vi "DPIO-Write Data.vi"(0 "DP stimulus params":T1={"Start (dB)"=0.0, "Stop (dB)"=0.0, "Step (dB)"=0.0, "Ear"=enum."Left", "Mode"=enum."L1 = L2", "f2 freqs (kHz)"=""}, 5 "AO Info":T3={"Samples/buffer (If continuous)"=10000, "p-p V output"=10.0, "Update Interval (uS)"=10, "# Reps"=10, "Mode"=0} {"Mode" items=["Free Run", "Set Reps", "WaveGen Only"]; "p-p V output" format="%.2f"}, 7 "DATA ARRAY TO SAVE":dbl[][](array[numeric])=[[60.0, 8337.40234375, 9997.55859375, 75.26988695602513, 60.02010719537736, -2.497224379667877, -6.035718747331266, -13.246407124310245, -10.010309675121785], [61.0, 8337.40234375, 9997.55859375, 75.26843338154123, 61.04772121995559, -10.079260881420453, -2.002824821632224, -13.478836216499538, -9.891536524361616], [62.0, 8337.40234375, 9997.55859375, 75.26842118127979, 62.07823756136253, -2.037295999935573, -2.3383554984418637, -7.356473706785984, -12.202574186674596], [63.0, 8337.40234375, 9997.55859375, 75.26689847125223, 63.11596204731964, 1.7137665521003527, -3.501789694558177, -12.430751170506419, -10.332402563871469], [64.0, 8337.40234375, 9997.55859375, 75.26410902438056, 64.14546808637438, 2.214385186705627, -2.5193547021211913, -13.192878839530465, -9.010065513616713], [65.0, 8337.40234375, 9997.55859375, 75.26244780852893, 65.23791090720081, 2.0929092941162324, -2.858976817533751, -9.447162706703264, -9.16426721329621], [66.0, 8337.40234375, 9997.55859375, 75.25853649879664, 66.25922378984633, 1.2609285848979752, -0.7601294228255071, -5.149516176783557, -11.823646373895414], [67.0, 8337.40234375, 9997.55859375, 75.25746587316436, 67.30068235725267, 2.1908463904635838, -2.0222825519681606, -4.18117048366198, -11.637986568273387], [68.0, 8337.40234375, 9997.55859375, 75.27653659482075, 68.25845427744406, -0.29516344046096776, -4.10442801745323, -4.280981245973685, -12.110717739994087], [69.0, 8337.40234375, 9997.55859375, 75.27405688750105, 69.30238527627466, -7.496556220976231, -3.7432906885060433, -6.52360859523705, -11.301872512577514], [70.0, 8337.40234375, 9997.55859375, 75.27095405136916, 70.32073725195177, -7.652753711444348, -2.8528280454442765, -12.182093372567518, -10.666926947025527], [71.0, 8337.40234375, 9997.55859375, 75.26930497101785, 71.37084081139689, -1.5072623443189102, -3.405227655422884, -9.054202292188972, -11.053257216259539], [72.0, 8337.40234375, 9997.55859375, 75.26969080860029, 72.40219775773258, -0.3774238902284708, -3.754108910689375, -6.28964062573494, -13.220161518942938], [73.0, 8337.40234375, 9997.55859375, 75.27097215908172, 73.44142356983946, -3.2633324671698247, -2.5245927600519877, -2.7612590826062373, -9.965708629780178], [74.0, 8337.40234375, 9997.55859375, 75.26718617542848, 74.4794351336158, -1.320663115916176, -4.039221123608023, -2.1363104698355713, -10.603442564638495], [75.0, 8337.40234375, 9997.55859375, 75.26504354514502, 75.52130171920129, -2.818101467950008, -3.4587578575361917, -6.091970124277275, -11.100841890245615]] format="%.2f", 9 "WAVEFORM ARRAY TO SAVE":dbl[][](array[numeric]) format="%.2f", 11 "error in (no error)":errorcluster, 12 "Averaging Specs":T4={"#Waves to Ave"=25, "#Spectra to Ave"=4}, 13 "Gain (dB)":dbl, 14 "Notes":string) -> (15 "error out":errorcluster)   [LabVIEW 2020]
uses:
  ABI Chamber VIs/LV Source/ABI Chamber Controller/SubVIs/ABI Globals.vi
  Utility VIs/Type Defs/Left-Right ring.ctl
  Typedefs/DP Stimulus Params.ctl
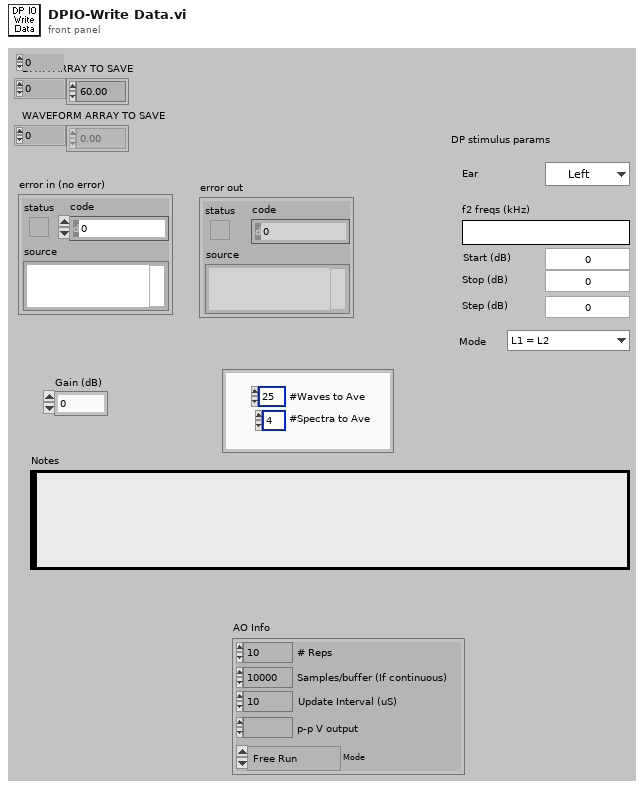
[diagram p1: front panel]
types:
  T1 = typedef "DP Stimulus Params.ctl" = cluster{"Start (dB)":dbl, "Stop (dB)":dbl, "Step (dB)":dbl, "Ear":T2, "Mode":enum16{"L1 = L2", "L1 = L2 + 10 dB"}, "f2 freqs (kHz)":string}
  T2 = typedef "Left-Right ring.ctl" = enum16{"Right", "Left"}
  T3 = cluster{"Samples/buffer (If continuous)":i32, "p-p V output":ext, "Update Interval (uS)":i32, "# Reps":i32, "Mode":u16}
  T4 = cluster{"#Waves to Ave":i32, "#Spectra to Ave":i32}
  T5 = enum16{"open", "replace", "create", "open or create", "replace or create", "replace or create with confirmation"}
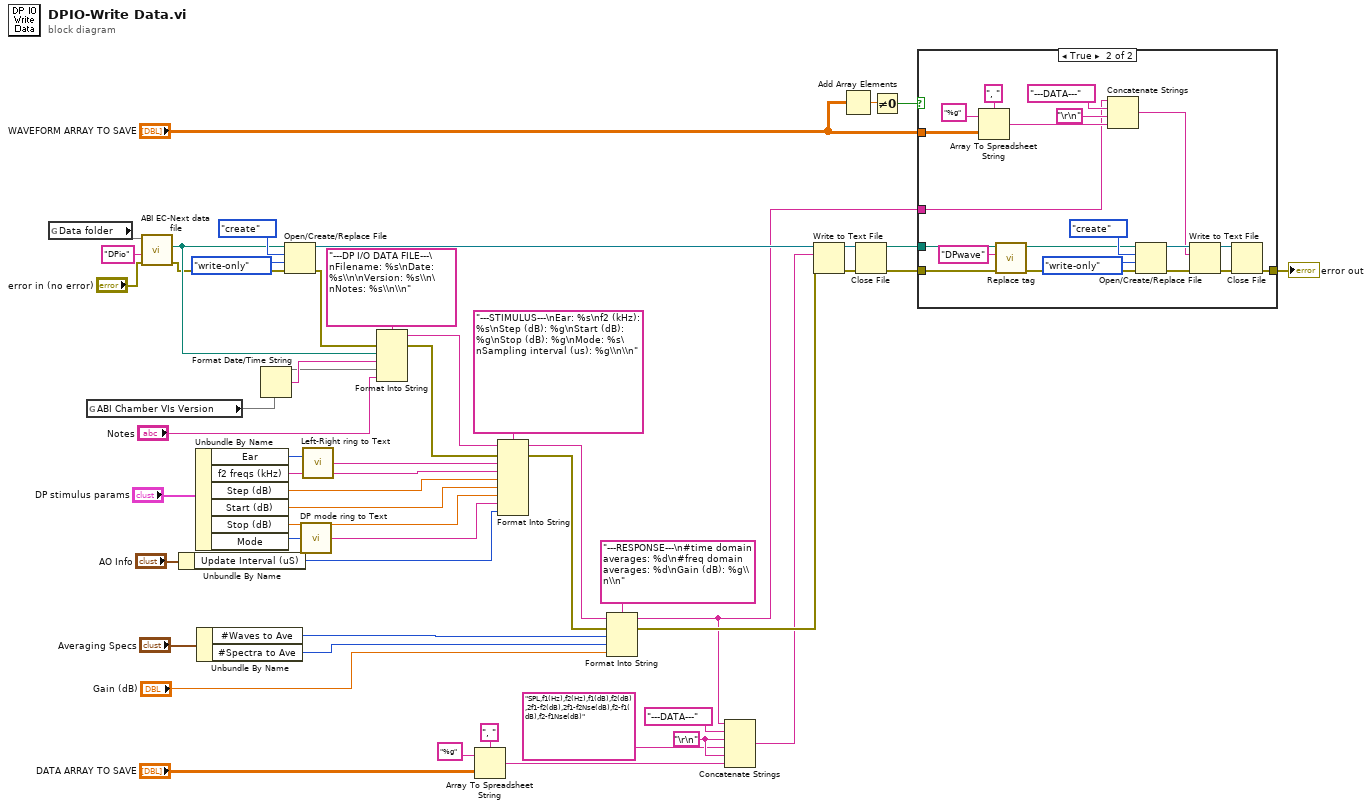
[diagram p0: block diagram]
diagram:
  w18 = "\r\n"
  n1 = global read "ABI Globals.vi" "Data folder"() -> (w15)
  n2 = global read "ABI Globals.vi" "ABI Chamber VIs Version"() -> (w31)
  n3 = call "ABI EC-Next data file.vi"("error in (no error)"="error in (no error)", "tag"="DPio", "Data folder"=w15) -> ("error IO"=w12:errorcluster, "dup path"=w14:path)  [unwired: 6 in, 1 out]
  n4 = Unbundle By Name("AO Info") -> ("Update Interval (uS)"=w41:i32)
  n5 = Unbundle By Name("DP stimulus params") -> ("Ear"=w40:T2, "f2 freqs (kHz)"=w38:string, "Step (dB)"=w37:dbl, "Start (dB)"=w36:dbl, "Stop (dB)"=w35:dbl, "Mode"=w25:enum16{"L1 = L2", "L1 = L2 + 10 dB"})
  n6 = Unbundle By Name("Averaging Specs") -> ("#Waves to Ave"=w29:i32, "#Spectra to Ave"=w28:i32)
  n7 = Format Date/Time String() -> (date/time string=w46:string)  [unwired: 3 in]
  n8 = Open/Create/Replace File(file path (use dialog)=w14, error in=w12, operation (0:open)=T5."create", access (0:read/write)=enum16{"read/write", "read-only", "write-only"}."write-only") -> (refnum out=w27:refnum<file>, error out=w45:errorcluster)  [unwired: 2 in, 1 out]
  n9 = call "DP mode ring to Text.vi"("Mode"=w25) -> ("Text"=w24:string)
  n10 = call "Left-Right ring to Text.vi"("Ear"=w40) -> ("Left/Right"=w39:string)
  n11 = Format Into String(format string="---DP I/O DATA FILE---\nFilename: %s\nDate: %s\\n\nVersion: %s\\n\nNotes: %s\\n\\n", error in=w45, w14, w46, w31, "Notes") -> (resulting string=w34:string, error out=w33:errorcluster)  [unwired: 1 in]
  n12 = Array To Spreadsheet String(delimiter (Tab)=", ", array="DATA ARRAY TO SAVE", 3:"%g" ("format string")) -> (spreadsheet string=w19:string)
  n13 = Format Into String(format string="---STIMULUS---\nEar: %s\nf2 (kHz): %s\nStep (dB): %g\nStart (dB): %g\nStop (dB): %g\nMode: %s\nSampling interval (us): %g\\n\\n", initial string=w34, error in=w33, w39, w38, w37, w36, w35, w24, w41) -> (resulting string=w1:string, error out=w2:errorcluster)
  n14 = Format Into String(format string="---RESPONSE---\n#time domain averages: %d\n#freq domain averages: %d\nGain (dB): %g\\n\\n", initial string=w1, error in=w2, w29, w28, "Gain (dB)") -> (resulting string=w3:string, error out=w26:errorcluster)
  n15 = Concatenate Strings(w3, "---DATA---" ("string"), w18, "SPL,f1(Hz),f2(Hz),f1(dB),f2(dB),2f1-f2(dB),2f1-f2Nse(dB),f2-f1(dB),f2-f1Nse(dB)", w18, w19) -> (w6:string)
  n16 = Write to Text File(file (use dialog)=w27, text=w6, error in=w26) -> (refnum out=w44:refnum<file>, error out=w43:errorcluster)  [unwired: 1 in, 1 out]
  n17 = Add Array Elements(numeric array="WAVEFORM ARRAY TO SAVE") -> (sum=w10:dbl)
  n18 = Close File(refnum=w44, error in=w43) -> (path=w8:path, error out=w5:errorcluster)
  n19 = Not Equal To 0?(x=w10) -> (x != 0?=w9:bool)
  n20 = case shown="True" w9 {
    tunnel: w8 -> [_ w58]
    tunnel: "WAVEFORM ARRAY TO SAVE" -> [_ w61]
    tunnel: w3 -> [_ w60]
    tunnel: w5 -> [w53 w57]
    tunnel: [w53 w67] -> w4
    frame False {
    }
    frame True {
      n21 = Array To Spreadsheet String(delimiter (Tab)=", ", array=w61, 3:"%g" ("format string")) -> (spreadsheet string=w63:string)
      n22 = call "Replace tag.vi"("error in (no error)"=w57, "tag"="DPwave", "Path"=w58) -> ("error out"=w56:errorcluster, "New Path"=w55:path)  [unwired: 7 in]
      n23 = Concatenate Strings(w60, "---DATA---" ("string"), "\r\n", w63) -> (w59:string)
      n24 = Open/Create/Replace File(file path (use dialog)=w55, error in=w56, operation (0:open)=T5."create", access (0:read/write)=enum16{"read/write", "read-only", "write-only"}."write-only") -> (refnum out=w69:refnum<file>, error out=w68:errorcluster)  [unwired: 2 in, 1 out]
      n25 = Write to Text File(file (use dialog)=w69, text=w59, error in=w68) -> (refnum out=w71:refnum<file>, error out=w70:errorcluster)  [unwired: 1 in, 1 out]
      n26 = Close File(refnum=w71, error in=w70) -> (error out=w67:errorcluster)  [unwired: 1 out]
    }
  }
  "error out" <- w4
